vi "StringComparison.vi"(9 "cmp":dbl, 10 "var":string, 11 "op":string) -> (3 "result":bool)   [LabVIEW 2011]
panel:
  in  "compares":T1(array[cluster])=[{"name"="NE", "op"=enum."ne"}, {"name"="EQ", "op"=enum."eq"}, {"name"="==", "op"=enum."eq"}, {"name"="!=", "op"=enum."ne"}, {"name"="GT", "op"=enum."gt"}, {"name"=">", "op"=enum."gt"}, {"name"="LT", "op"=enum."lt"}, {"name"="<", "op"=enum."lt"}, {"name"="LTEQ", "op"=enum."lteq"}, {"name"="<=", "op"=enum."lteq"}, {"name"="GTEQ", "op"=enum."gteq"}, {"name"=">=", "op"=enum."gteq"}]
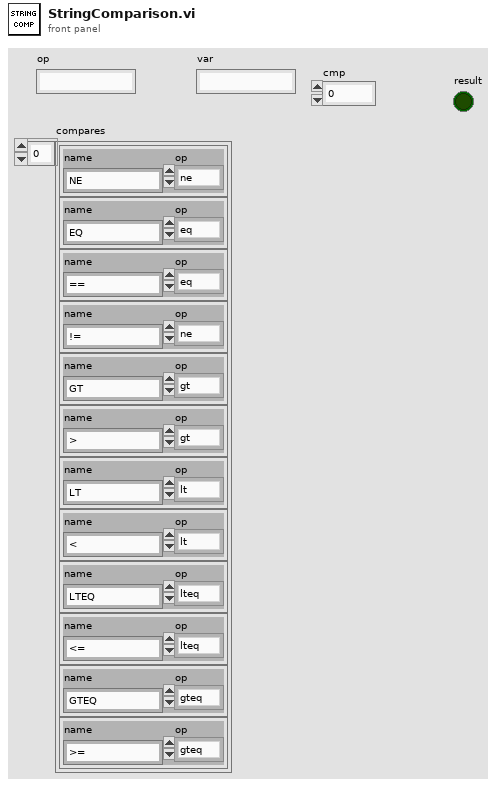
[diagram p1: front panel]
types:
  T1 = cluster{"name":string, "op":enum16{"eq", "ne", "lteq", "gteq", "lt", "gt"}}[]
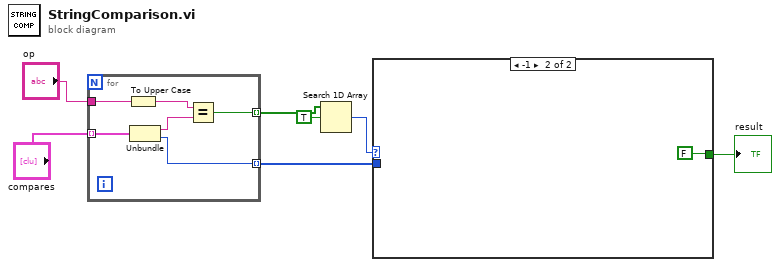
[diagram p0: block diagram]
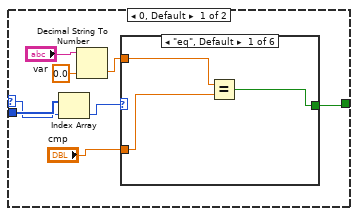
[diagram p2: hidden frame]
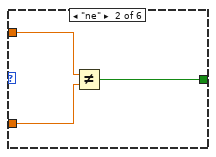
[diagram p3: hidden frame]
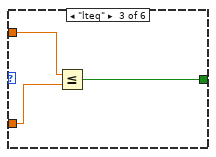
[diagram p4: hidden frame]
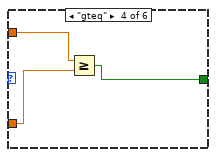
[diagram p5: hidden frame]
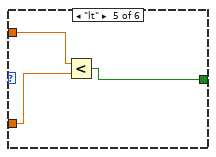
[diagram p6: hidden frame]
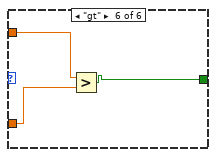
[diagram p7: hidden frame]
diagram:
  n1 = for {
    tunnel: "compares" -> [w13] mode=indexing
    tunnel: "op" -> [w12]
    tunnel: [w9] -> w5 mode=indexing
    tunnel: [w8] -> w1 mode=indexing
    n2 = To Upper Case(1:w12) -> (0:w11:string)
    n3 = Unbundle(w13) -> ("name"=w10:string, "op"=w8:enum16{"eq", "ne", "lteq", "gteq", "lt", "gt"})
    n4 = Equal?(x=w11, y=w10) -> (x = y?=w9:bool)
  }
  n5 = Search 1D Array(1D array=w5, element=TRUE) -> (index of element=w3:i32)  [unwired: 1 in]
  n6 = case shown="-1" w3 {
    selector: w3 -> [w20 _]
    tunnel: [w18 FALSE ("result")] -> w2
    tunnel: w1 -> [w21 _]
    frame 0, Default {
      n7 = Index Array(array=w21, index=w20) -> (element=w19:enum16{"eq", "ne", "lteq", "gteq", "lt", "gt"})
      n8 = Decimal String To Number(string="var", default (0L)=0.0 ("default (0 I32)")) -> (number=w15:dbl)  [unwired: 1 in, 1 out]
      n9 = case shown="\"eq\", Default" w19 {
        tunnel: w15 -> [w24 w27 w30 w33 w36 w39]
        tunnel: "cmp" -> [w23 w26 w29 w32 w35 w38]
        tunnel: [w22 w25 w28 w31 w34 w37] -> w18
        frame "eq", Default {
          n10 = Equal?(x=w24, y=w23) -> (x = y?=w22:bool)
        }
        frame "ne" {
          n11 = Not Equal?(x=w27, y=w26) -> (x != y?=w25:bool)
        }
        frame "lteq" {
          n12 = Less Or Equal?(x=w30, y=w29) -> (x <= y?=w28:bool)
        }
        frame "gteq" {
          n13 = Greater Or Equal?(x=w33, y=w32) -> (x >= y?=w31:bool)
        }
        frame "lt" {
          n14 = Less?(x=w36, y=w35) -> (x < y?=w34:bool)
        }
        frame "gt" {
          n15 = Greater?(x=w39, y=w38) -> (0:w37:bool)
        }
      }
    }
    frame -1 {
    }
  }
  "result" <- w2
